vi "Disconnect.vi"(8 "error in (no error)":errorcluster, 10 "Force (T)":bool=TRUE, 11 "PVConnection in":refnum<class "PVConnection.lvclass">) -> (0 "error out":errorcluster, 3 "PVConnection out":refnum<class "PVConnection.lvclass">)   [LabVIEW 2015, in "CS++ProcessVariables.lvlib" / "PVConnection.lvclass"]
doc: "Close reference to a process variable."
uses:
  PVConnection.lvclass
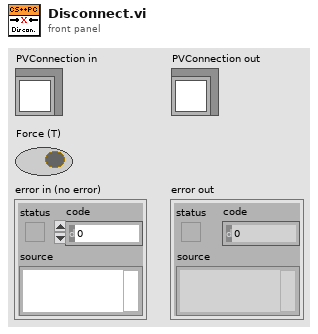
[diagram p1: front panel]
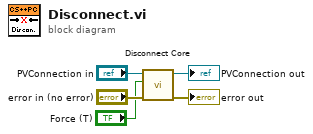
[diagram p0: block diagram]
diagram:
  n1 = call-dynamic "Disconnect Core.vi"("error in (no error)"="error in (no error)", "Force (T)"="Force (T)", "PVConnection in"="PVConnection in") -> ("error out"=→"error out":errorcluster, "PVConnection out"=→"PVConnection out":refnum<class "PVConnection.lvclass">)  [unwired: 7 in]
